vi "DiJian_write.vi"(7 "COM通道":u32=1, 8 "error in":errorcluster, 9 "地检2相位":i32, 10 "地检1相位":i32, 11 "VISA资源名称":refnum<visa-resource-name>) -> (0 "错误输出":errorcluster, 1 "地检2相位输出":i32, 2 "地检1相位输出":i32, 3 "VISA资源名称输出":refnum<visa-resource-name>)   [LabVIEW 2012]
uses:
  <vilib>/GPower/VIRegister/Library/Convert/ToDBL.vi
  <vilib>/GPower/VIRegister/Library/SubVIs/FindRegisterData.vi
  <vilib>/GPower/VIRegister/Library/SubVIs/ReadSub.vi
  <vilib>/GPower/VIRegister/Library/QManager/GetRegisterData.vi
  <vilib>/GPower/Error/Library/SetError.vi
  <vilib>/GPower/Error/Library/FilterCodes.vi
  <vilib>/GPower/Error/Library/Filter/FilterMulti.vi
  <vilib>/GPower/VIRegister/Library/QManager/QManagerAction.vi
  <vilib>/GPower/Error/Library/ErrorType.vi
  <vilib>/GPower/Error/Library/SplitAppended.vi
  <vilib>/GPower/Error/Library/SubVIs/ExplanationToError.vi
  <vilib>/GPower/VIRegister/Library/QManager/GetQName.vi
  <vilib>/GPower/VIRegister/Library/QManager/StartQManager.vi
  <vilib>/Utility/error.llb/Trim Whitespace.vi
  <vilib>/dlg_ctls.llb/Space Constant.vi
  <vilib>/Utility/error.llb/Error Code Database.vi
  <vilib>/GPower/Error/Library/SubVIs/SetStatus.vi
  <vilib>/GPower/Error/Library/AppendErrors.vi
  <vilib>/GPower/Error/Library/Append/AppendSingle.vi
  com/TONGXUN/write32.vi
  <vilib>/GPower/VIRegister/VIRegister.lvlib
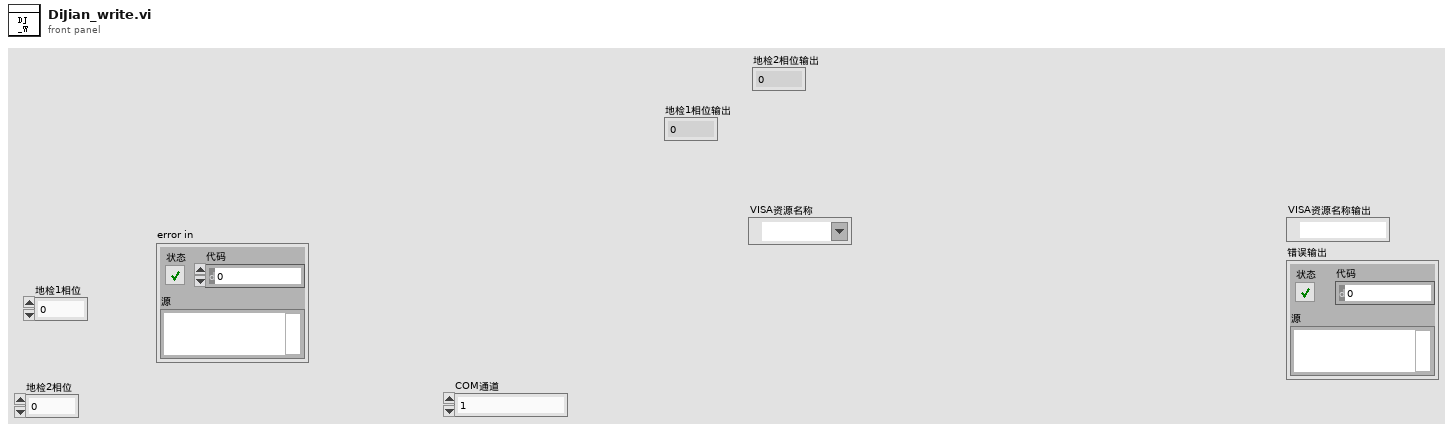
[diagram p1: front panel]
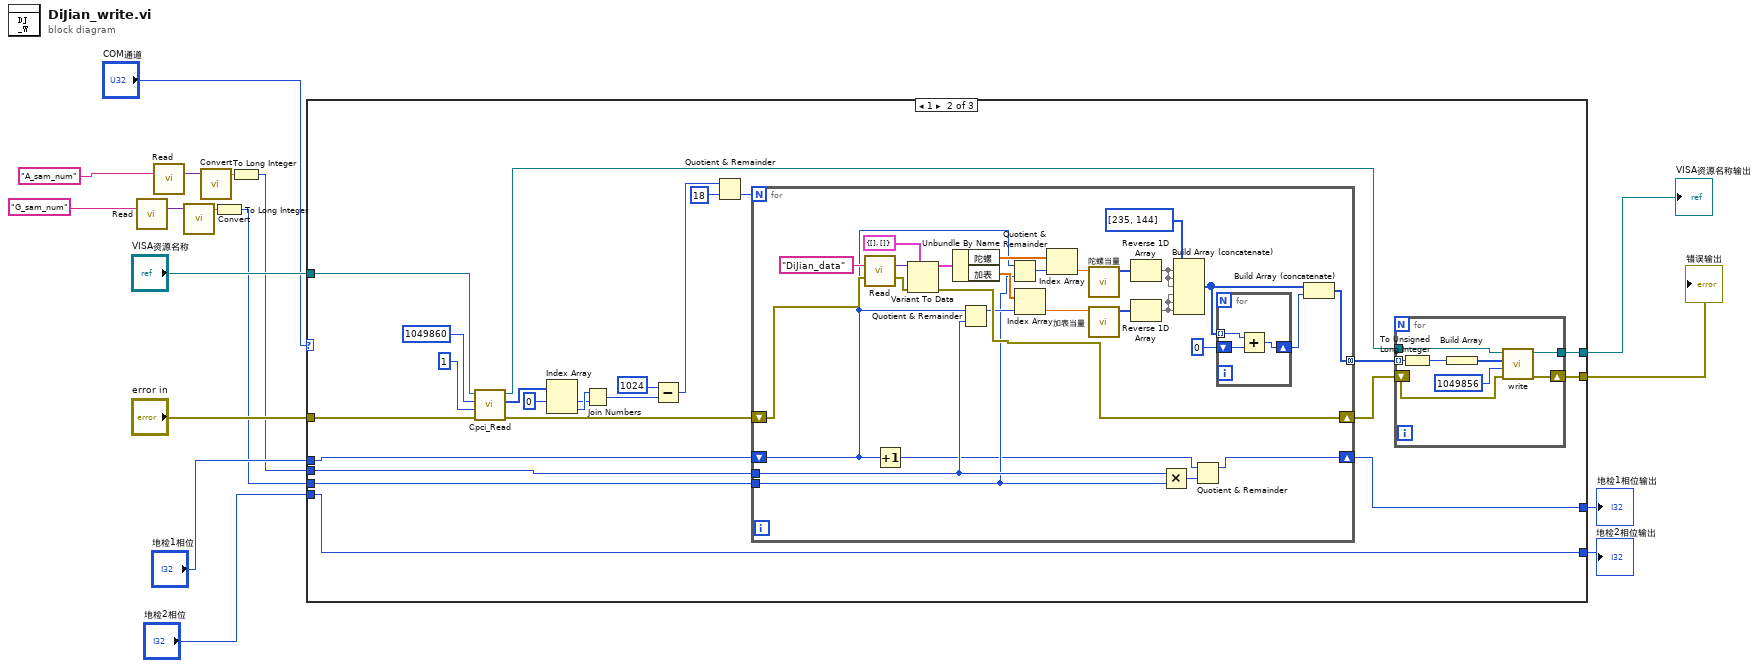
[diagram p0: block diagram]
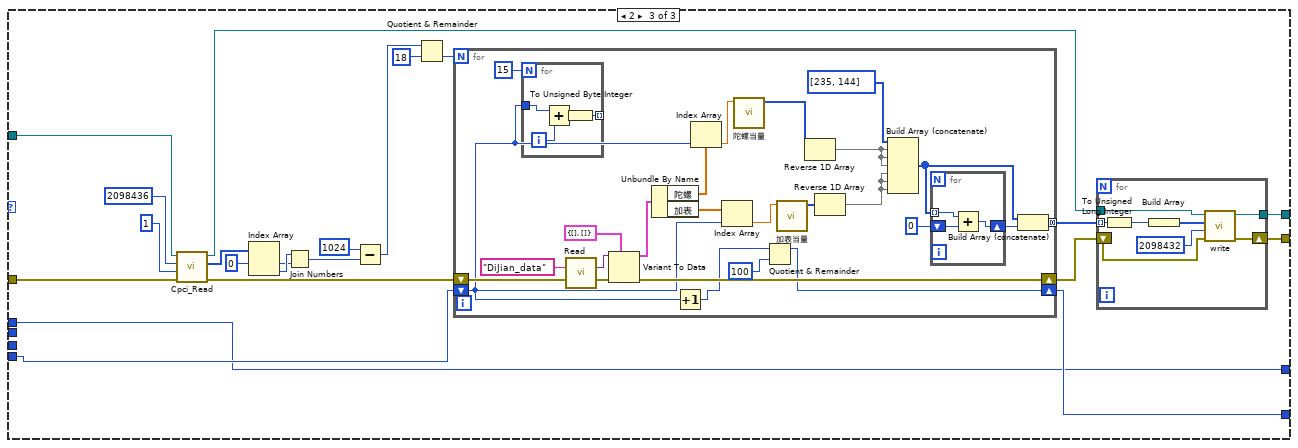
[diagram p3: hidden frame]
diagram:
  n1 = call <vilib>:"Read.vi"("Register name"="G_sam_num") -> ("Register value"=w4:variant)  [unwired: 11 in, 3 out]
  n2 = call <vilib>:"Read.vi"("Register name"="A_sam_num") -> ("Register value"=w7:variant)  [unwired: 11 in, 3 out]
  n3 = call-poly <vilib>:"Convert.vi"("Register value in"=w4) -> ("Register value out"=w3:dbl)  [unwired: 13 in, 1 out]
  n4 = call-poly <vilib>:"Convert.vi"("Register value in"=w7) -> ("Register value out"=w8:dbl)  [unwired: 13 in, 1 out]
  n5 = To Long Integer(number=w3) -> (32bit integer=w1:i32)
  n6 = To Long Integer(number=w8) -> (32bit integer=w5:i32)
  n7 = case shown="1" "COM通道" {
    tunnel: "VISA资源名称" -> [w21 w33 w94]
    tunnel: [w21 w31 w92] -> w16
    tunnel: "error in" -> [w20 w29 w90]
    tunnel: [w20 w27 w88] -> w14
    tunnel: "地检2相位" -> [w19 w24 w87]
    tunnel: "地检1相位" -> [w18 w26 w85]
    tunnel: [w18 w25 w85] -> w10
    tunnel: [w19 w24 w86] -> w9
    tunnel: w5 -> [_ w23 _]
    tunnel: w1 -> [_ w22 _]
    frame 0, Default {
    }
    frame 1 {
      n8 = call "Cpci_Read.vi"("错误输入（无错误）"=w29, "u32_len"=1, "基地址"=u32 1049860, "VISA资源名称"=w33) -> ("错误输出"=w28:errorcluster, "U8"=w39:u8[], "VISA资源名称输出"=w32:refnum<visa-resource-name>)  [unwired: 5 in]
      n9 = Index Array(array=w39, index #1=0 ("索引")) -> (element #1=w36:u8, element #2=w37:u8)  [unwired: 1 in]
      n10 = Join Numbers(hi=w37, lo=w36) -> ((hi.lo)=w42:u16)
      n11 = Subtract(x=u16 1024, y=w42) -> (x-y=w44:u16)
      n12 = Quotient & Remainder(x=w44, y=u16 18) -> (floor(x/y)=w35:u16)  [unwired: 1 out]
      n13 = for {
        N: w35 -> [_]
        tunnel: [w72] -> w34 mode=concatenating
        shift-right: [w71] -> w30
        shift-left: w28 -> [w70]
        shift-right: [w56] -> w25
        shift-left: w26 -> [w54]
        tunnel: w23 -> [w59]
        tunnel: w22 -> [w58]
        n14 = call <vilib>:"Read.vi"("Register name"="DiJian_data", "Error in"=w70) -> ("Register value"=w78:variant, "Error out"=w74:errorcluster)  [unwired: 10 in, 2 out]
        n15 = Increment(x=w54) -> (x+1=w55:i32)
        n16 = Variant To Data(error in=w74, type=cluster{"陀螺":dbl[], "加表":dbl[]} {"陀螺"=[], "加表"=[]} ("输入簇"), Variant=w78) -> (data=w79:cluster{"陀螺":dbl[], "加表":dbl[]}, error out=w71:errorcluster)
        n17 = Unbundle By Name(w79) -> ("陀螺"=w80:dbl[], "加表"=w81:dbl[])
        n18 = Quotient & Remainder(x=w54, y=w59) -> (x-y*floor(x/y)=w60:i32)  [unwired: 1 out]
        n19 = Quotient & Remainder(x=w54, y=w58) -> (x-y*floor(x/y)=w61:i32)  [unwired: 1 out]
        n20 = Index Array(array=w81, index=w60) -> (element=w66:dbl)
        n21 = Index Array(array=w80, index=w61) -> (element=w68:dbl)
        n22 = call "陀螺当量.vi"("x"=w68) -> ("子数组"=w67:u8[])  [unwired: 10 in]
        n23 = call "加表当量.vi"("x"=w66) -> ("子数组"=w65:u8[])  [unwired: 10 in]
        n24 = Reverse 1D Array(array=w67) -> (reversed array=w63:u8[])
        n25 = Reverse 1D Array(array=w65) -> (reversed array=w62:u8[])
        n26 = Multiply(x=w59, y=w58) -> (x*y=w57:i32)
        n27 = Build Array (concatenate)(u8[] [235, 144] ("数组"), w63, w63, w63, w62, w62, w62) -> (w64:u8[])
        n28 = Quotient & Remainder(x=w55, y=w57) -> (x-y*floor(x/y)=w56:i32)  [unwired: 1 out]
        n29 = for {
          tunnel: w64 -> [w84] mode=indexing
          shift-right: [w82] -> w75
          shift-left: u8 0 ("y") -> [w83]
          n30 = Add(x=w84, y=w83) -> (x+y=w82:u8)
        }
        n31 = Build Array (concatenate)(w64, w75) -> (w72:u8[])
      }
      n32 = for {
        tunnel: w34 -> [w53] mode=indexing
        tunnel: w32 -> [w52]
        tunnel: [w51] -> w31
        shift-right: [w49] -> w27
        shift-left: w30 -> [w50]
        n33 = To Unsigned Long Integer(number=w53) -> (unsigned 32bit integer=w46:u32)
        n34 = Build Array(w46) -> (w47:u32[])
        n35 = call-poly "write.vi"("error out"=w50, "起始地址"=u32 1049856, "U32"=w47, "VISA资源名称输入"=w52) -> ("error out 2"=w49:errorcluster, "VISA资源名称输出"=w51:refnum<visa-resource-name>)  [unwired: 6 in]
      }
    }
    frame 2 {
      n36 = call "Cpci_Read.vi"("错误输入（无错误）"=w90, "u32_len"=1, "基地址"=u32 2098436, "VISA资源名称"=w94) -> ("错误输出"=w89:errorcluster, "U8"=w100:u8[], "VISA资源名称输出"=w93:refnum<visa-resource-name>)  [unwired: 5 in]
      n37 = Index Array(array=w100, index #1=0 ("索引")) -> (element #1=w97:u8, element #2=w98:u8)  [unwired: 1 in]
      n38 = Join Numbers(hi=w98, lo=w97) -> ((hi.lo)=w103:u16)
      n39 = Subtract(x=u16 1024, y=w103) -> (x-y=w105:u16)
      n40 = Quotient & Remainder(x=w105, y=u16 18) -> (floor(x/y)=w96:u16)  [unwired: 1 out]
      n41 = for {
        N: w96 -> [_]
        tunnel: [w130] -> w95 mode=concatenating
        shift-right: [w129] -> w91
        shift-left: w89 -> [w128]
        shift-right: [w125] -> w86
        shift-left: w87 -> [w123]
        n42 = for {
          N: 15 -> [_]
          tunnel: w123 -> [w143]
          tunnel: [w140] -> _ mode=indexing
          i -> [w142]
          n43 = Add(x=w143, y=w142) -> (x+y=w141:i32)
          n44 = To Unsigned Byte Integer(number=w141) -> (unsigned 8bit integer=w140:u8)
        }
        n45 = call <vilib>:"Read.vi"("Register name"="DiJian_data", "Error in"=w128) -> ("Register value"=w136:variant, "Error out"=w132:errorcluster)  [unwired: 10 in, 2 out]
        n46 = Variant To Data(error in=w132, type=cluster{"陀螺":dbl[], "加表":dbl[]} {"陀螺"=[], "加表"=[]} ("输入簇"), Variant=w136) -> (data=w137:cluster{"陀螺":dbl[], "加表":dbl[]}, error out=w129:errorcluster)
        n47 = Unbundle By Name(w137) -> ("陀螺"=w138:dbl[], "加表"=w139:dbl[])
        n48 = Increment(x=w123) -> (x+1=w126:i32)
        n49 = Index Array(array=w138, index=w123) -> (element=w121:dbl)
        n50 = Index Array(array=w139, index=w123) -> (element=w119:dbl)
        n51 = call "陀螺当量.vi"("x"=w121) -> ("子数组"=w120:u8[])  [unwired: 10 in]
        n52 = Quotient & Remainder(x=w126, y=100) -> (x-y*floor(x/y)=w125:i32)  [unwired: 1 out]
        n53 = call "加表当量.vi"("x"=w119) -> ("子数组"=w118:u8[])  [unwired: 10 in]
        n54 = Reverse 1D Array(array=w120) -> (reversed array=w116:u8[])
        n55 = Reverse 1D Array(array=w118) -> (reversed array=w115:u8[])
        n56 = Build Array (concatenate)(u8[] [235, 144] ("数组"), w116, w116, w116, w115, w115, w115) -> (w117:u8[])
        n57 = for {
          tunnel: w117 -> [w146] mode=indexing
          shift-right: [w144] -> w133
          shift-left: u8 0 ("y") -> [w145]
          n58 = Add(x=w146, y=w145) -> (x+y=w144:u8)
        }
        n59 = Build Array (concatenate)(w117, w133) -> (w130:u8[])
      }
      n60 = for {
        tunnel: w95 -> [w114] mode=indexing
        tunnel: w93 -> [w113]
        tunnel: [w112] -> w92
        shift-right: [w110] -> w88
        shift-left: w91 -> [w111]
        n61 = To Unsigned Long Integer(number=w114) -> (unsigned 32bit integer=w107:u32)
        n62 = Build Array(w107) -> (w108:u32[])
        n63 = call-poly "write.vi"("error out"=w111, "起始地址"=u32 2098432, "U32"=w108, "VISA资源名称输入"=w113) -> ("error out 2"=w110:errorcluster, "VISA资源名称输出"=w112:refnum<visa-resource-name>)  [unwired: 6 in]
      }
    }
  }
  "VISA资源名称输出" <- w16
  "错误输出" <- w14
  "地检1相位输出" <- w10
  "地检2相位输出" <- w9
